vi "Client - STOP ALL Actors.vi"(8 "error in":errorcluster) -> (0 "error out":errorcluster)   [LabVIEW 2023, in "Client.lvlib" / "Client.lvclass"]
uses:
  Client.lvclass
  Client - Ctrl - FGV - Action.ctl
  <vilib>/ActorFramework/Stop Msg/Stop Msg.lvclass
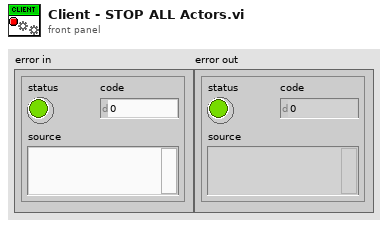
[diagram p1: front panel]
types:
  T1 = typedef "Client.lvlib/Client.lvclass/Client - Ctrl - FGV - Action.ctl" = enum16{"Int", "Get"}
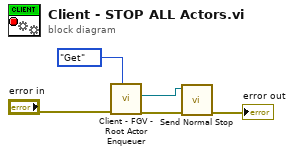
[diagram p0: block diagram]
diagram:
  n1 = call "Client - FGV - Root Actor Enqueuer.vi"("Action"=Client_-_Ctrl_-_FGV_-_Action."Get", "error in"="error in") -> ("error out"=w4:errorcluster, "Root Enqueuer"=w3:refnum<class "Message Enqueuer.lvclass">)  [unwired: 8 in]
  n2 = call <vilib>:"Send Normal Stop.vi"("error in (no error)"=w4, "Message Enqueuer"=w3) -> ("error out"=→"error out":errorcluster)  [unwired: 9 in]
